vi "Refgroup.vi"(6 "Pane":refnum<vi>, 7 "Action":enum16{"GetRef", "ChkRef"}(ring)) -> (0 "AreaSize":T1, 1 "Ref_Gmsg":refnum<vi>, 2 "Ref_Ball":refnum<vi>, 3 "Ref_brick":refnum<vi>[](array[refnum]))   [LabVIEW 2014]
uses:
  <vilib>/Utility/miscctls.llb/LVBoundsTypeDef.ctl
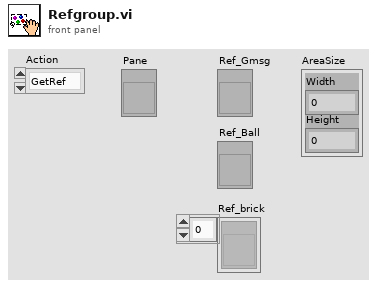
[diagram p1: front panel]
types:
  T1 = typedef "LVBoundsTypeDef.ctl" = cluster{"Width":u32, "Height":u32}
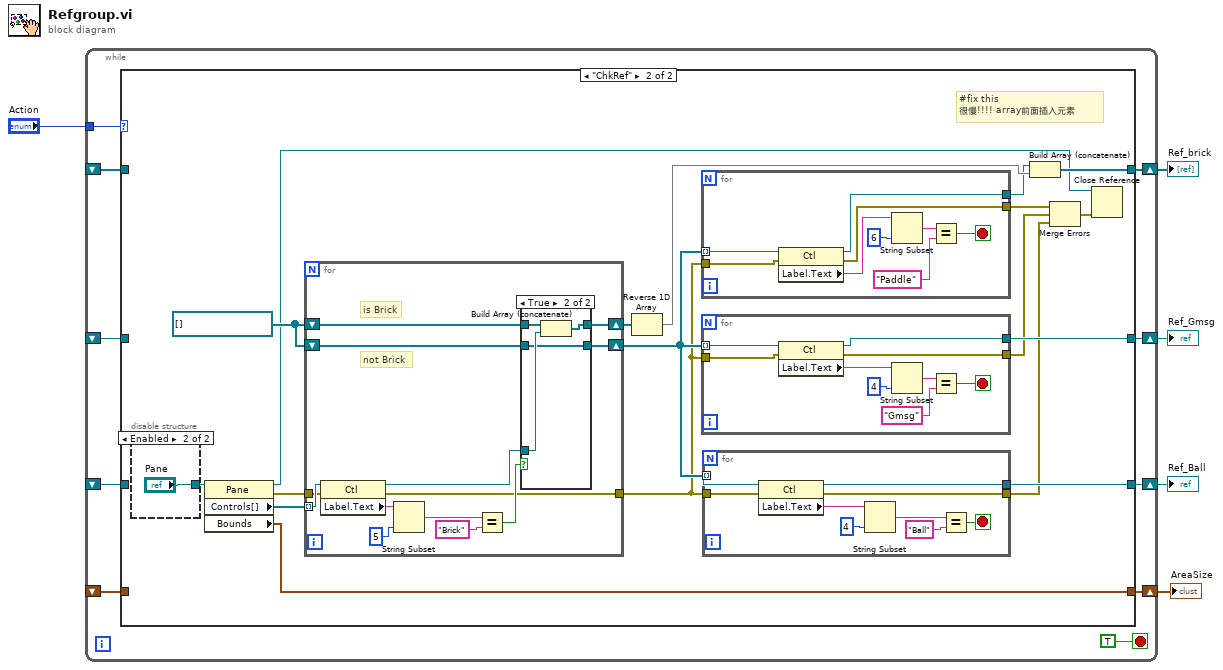
[diagram p0: block diagram]
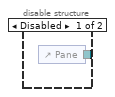
[diagram p3: hidden frame]
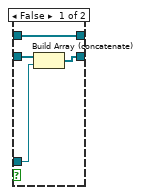
[diagram p4: hidden frame]
diagram:
  n1 = while {
    shift-right: [w12] -> w2
    shift-left: _ -> [w6]
    shift-right: [w15] -> w5
    shift-left: _ -> [w8]
    shift-right: [w14] -> w4
    shift-left: _ -> [w7]
    shift-right: [w13] -> w3
    shift-left: _ -> [w9]
    tunnel: "Action" -> [w10]
    stop <- TRUE stop-if-true
    n2 = case shown="\"ChkRef\"" w10 {
      tunnel: [w18 w35] -> w15
      tunnel: [w17 w34] -> w14
      tunnel: [w19 w33] -> w13
      tunnel: [w16 w32] -> w12
      tunnel: w9 -> [w19 _]
      tunnel: w8 -> [w18 _]
      tunnel: w7 -> [w17 _]
      tunnel: w6 -> [w16 _]
      frame "GetRef", Default {
      }
      frame "ChkRef" {
        w31 = refnum<vi>[] []
        # "#fix this\n很慢!!!! array前面插入元素"
        n3 = disable-structure shown="Enabled" {
          disable-tunnel: [w38 "Pane"] -> w37
          frame Disabled {
            n4 = control-ref of="Pane"() -> (w38:refnum<vi>)
          }
          frame Enabled {
          }
        }
        n5 = property class="Pane"(reference=w37) -> (reference out=w26:refnum<vi>, error out=w28:errorcluster, "Controls[]"=w30:refnum<vi>[], "Bounds"=w32:T1)  [unwired: 1 in]
        n6 = for {
          shift-right: [w74] -> w36
          shift-left: w31 -> [w75]
          tunnel: [w72] -> w27
          shift-right: [w70] -> w29
          shift-left: w31 -> [w69]
          tunnel: w30 -> [w68] mode=indexing
          tunnel: w28 -> [w67]
          # "not Brick"
          # "is Brick"
          n7 = property on="Property Node" class="Ctl"(reference=w68, error in=w67) -> (reference out=w71:refnum<vi>, error out=w72:errorcluster, "Label.Text"=w73:string)
          n8 = String Subset(string=w73, length (rest)=5 ("length (rest)")) -> (substring=w77:string)  [unwired: 1 in]
          n9 = Equal?(x=w77, y="Brick") -> (x = y?=w76:bool)
          n10 = case shown="True" w76 {
            tunnel: w75 -> [w83 w86]
            tunnel: [w83 w87] -> w74
            tunnel: w71 -> [w82 w85]
            tunnel: [w81 w84] -> w70
            tunnel: w69 -> [w80 w84]
            frame False {
              n11 = Build Array (concatenate)(w80, w82) -> (w81:refnum<vi>[])
            }
            frame True {
              n12 = Build Array (concatenate)(w86, w85) -> (w87:refnum<vi>[])
            }
          }
        }
        n13 = Reverse 1D Array(array=w36) -> (reversed array=w21:refnum<vi>[])
        n14 = for {
          tunnel: [w44] -> w24
          tunnel: [w42] -> w20
          tunnel: w29 -> [w41] mode=indexing
          tunnel: w27 -> [w40]
          stop <- w43 stop-if-true
          n15 = property on="Property Node" class="Ctl"(reference=w41, error in=w40) -> (reference out=w42:refnum<vi>, error out=w44:errorcluster, "Label.Text"=w48:string)
          n16 = String Subset(string=w48, length (rest)=6 ("length (rest)")) -> (substring=w47:string)  [unwired: 1 in]
          n17 = Equal?(x=w47, y="Paddle") -> (x = y?=w43:bool)
        }
        n18 = for {
          tunnel: [w61] -> w35
          tunnel: [w60] -> w22
          tunnel: w29 -> [w59] mode=indexing
          tunnel: w27 -> [w58]
          stop <- w62 stop-if-true
          n19 = property on="Property Node" class="Ctl"(reference=w59, error in=w58) -> (reference out=w61:refnum<vi>, error out=w60:errorcluster, "Label.Text"=w66:string)
          n20 = String Subset(string=w66, length (rest)=4 ("length (rest)")) -> (substring=w65:string)  [unwired: 1 in]
          n21 = Equal?(x=w65, y="Gmsg") -> (x = y?=w62:bool)
        }
        n22 = for {
          tunnel: [w53] -> w34
          tunnel: [w52] -> w23
          tunnel: w29 -> [w50] mode=indexing
          tunnel: w27 -> [w49]
          stop <- w51 stop-if-true
          n23 = property on="Property Node" class="Ctl"(reference=w50, error in=w49) -> (reference out=w53:refnum<vi>, error out=w52:errorcluster, "Label.Text"=w54:string)
          n24 = String Subset(string=w54, length (rest)=4 ("length (rest)")) -> (substring=w55:string)  [unwired: 1 in]
          n25 = Equal?(x=w55, y="Ball") -> (x = y?=w51:bool)
        }
        n26 = Build Array (concatenate)(w20, w21) -> (w33:refnum<vi>[])
        n27 = Merge Errors(w24, w22, w23) -> (w25:errorcluster)
        n28 = Close Reference(reference=w26, error in (no error)=w25) -> ()  [unwired: 1 out]
      }
    }
  }
  "Ref_Gmsg" <- w5
  "Ref_Ball" <- w4
  "Ref_brick" <- w3
  "AreaSize" <- w2
